vi "Main.vi"() -> ()   [LabVIEW 2020]
uses:
  Typedef/Processs.ctl
  Typedef/Low Ingregians.ctl
  Typedef/Quanities.ctl
  Assignment 14/Car Wash/CarWash/Typedefs/Queue Operations.ctl
  Typedef/DataCluster.ctl
  <vilib>/Utility/config.llb/Read Key (Boolean).vi
  <vilib>/Utility/config.llb/Write Key (Boolean).vi
  <vilib>/Utility/config.llb/NI_LVConfig.lvlib
panel:
  in  "Quantity":T1
  out "Low Ingredian":T2
  out "Process":T3
  in  "Power":bool
  out "Error Out":errorcluster
  in  "Error In":errorcluster
  out "Total Cups":dbl
  out "Elapsed Time":dbl
  out "Dispenser":dbl(slide) scale=0.0..60.0
  out "Chamber":dbl(slide) scale=0.0..60.0
  in  "Knob":i32(knob) scale=0.0..2.0
  out "Milk Level":dbl(slide)=100.0 scale=0.0..100.0
  out "Bean Level":dbl(slide)=100.0 scale=0.0..100.0
  out "Water Level":dbl(slide)=100.0 scale=0.0..100.0
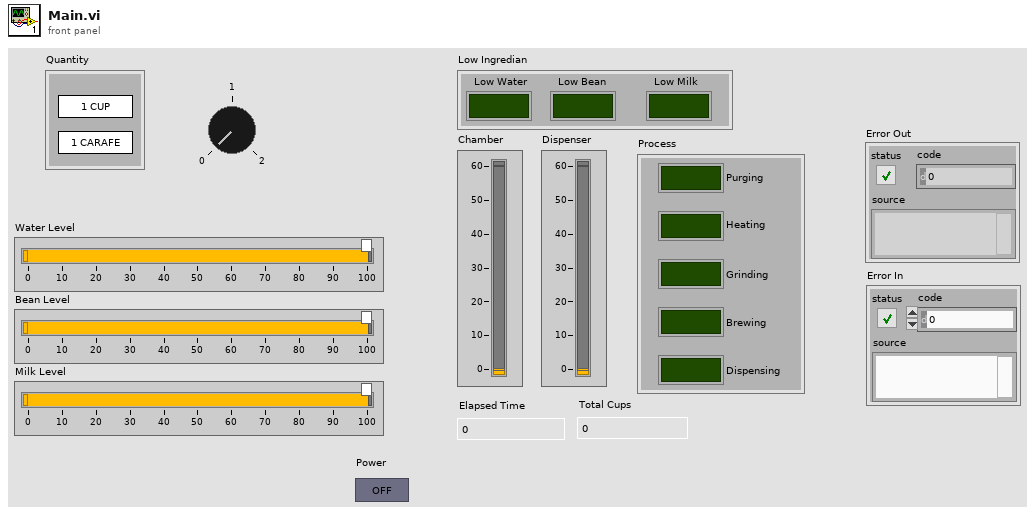
[diagram p1: front panel]
types:
  T1 = typedef "Quanities.ctl" = cluster{"1 Carafe":bool, "1 Cup":bool}
  T2 = typedef "Low Ingregians.ctl" = cluster{"Low Water":bool, "Low Bean":bool, "Low Milk":bool}
  T3 = typedef "Processs.ctl" = cluster{"Purging":bool, "Heating":bool, "Grinding":bool, "Brewing":bool, "Dispensing":bool}
  T4 = typedef "DataCluster.ctl" = cluster{"Water Level":dbl, "Bean Level":dbl, "Milk Level":dbl, "Knob":i32, "Chamber":dbl, "Dispenser":dbl, "Elapsed Time":dbl, "Total Cups":dbl, "Timer":cluster{"Previous Time":dbl, "Elapsed Time":dbl, "Start":bool, "Pause":bool, "Set Time":dbl}, "Sequence Data":i32, "Sequence":string[], "Quantity":T1, "Low Ingredian":T2, "Process":T3, "Enable array":refnum<vi>[], "Disable array":refnum<vi>[], "Power ":bool}
  T5 = typedef "Queue Operations.ctl" = enum16{"Create", "Enqueue", "Enqueue N elements", "Enstack", "Enstack N elements", "Dequeue", "Flush queue", "Release queue"}
  T6 = typedef "NI_LVConfig.lvlib/Config Data RefNum.ctl" = refnum<k1>
  T7 = enum8{"Enabled", "Disabled", "Disabled and Grayed Out"}
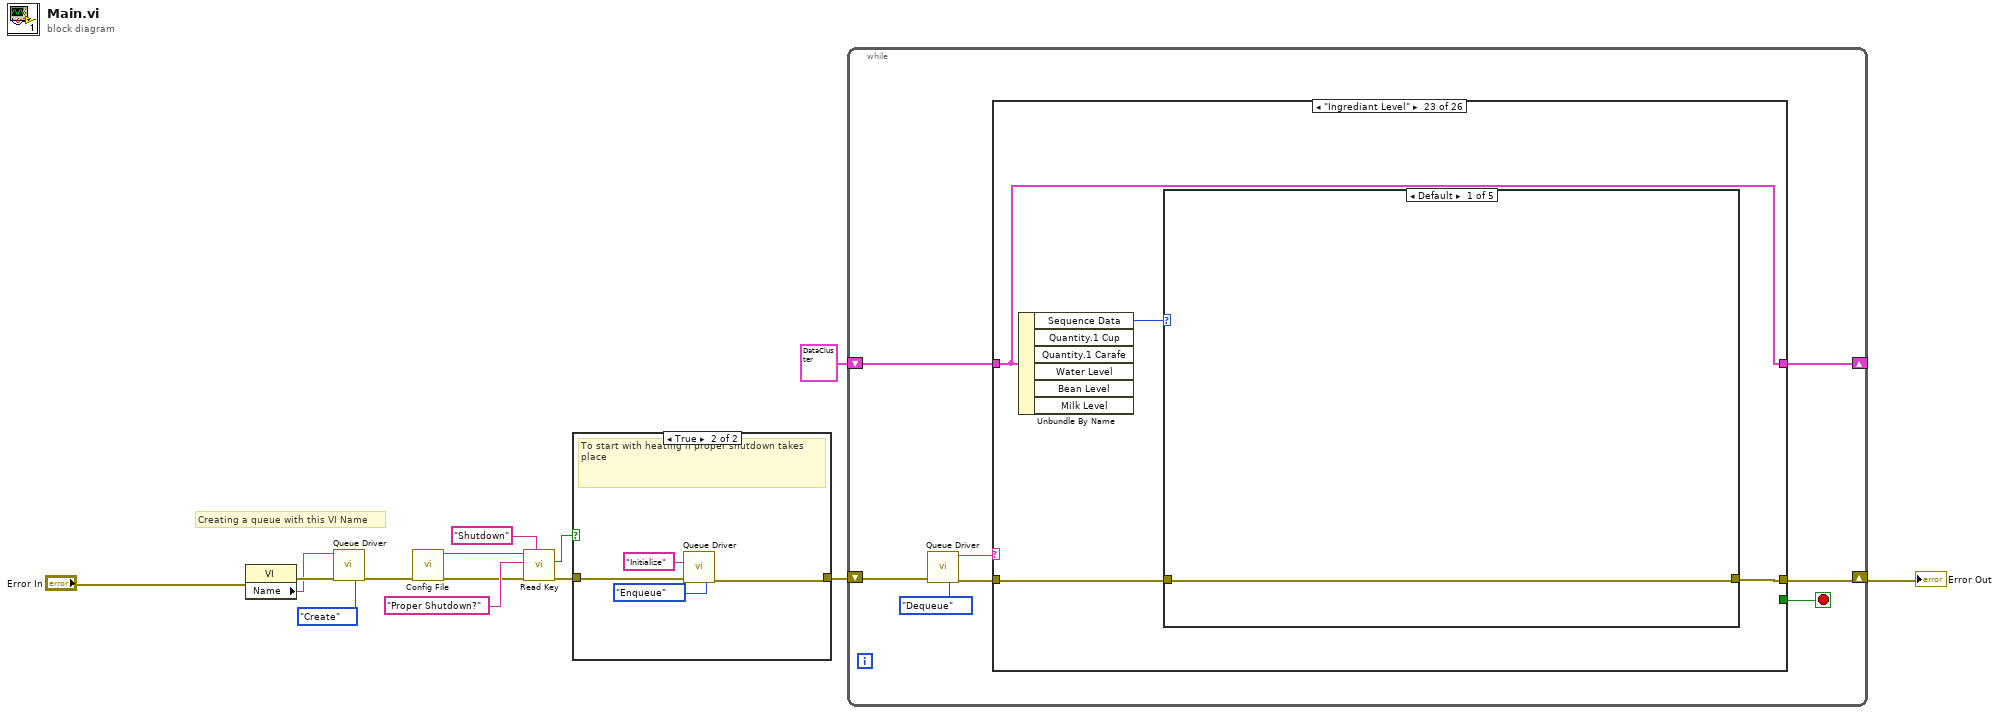
[diagram p0: block diagram]
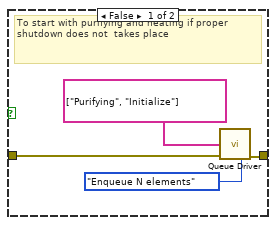
[diagram p2: hidden frame]
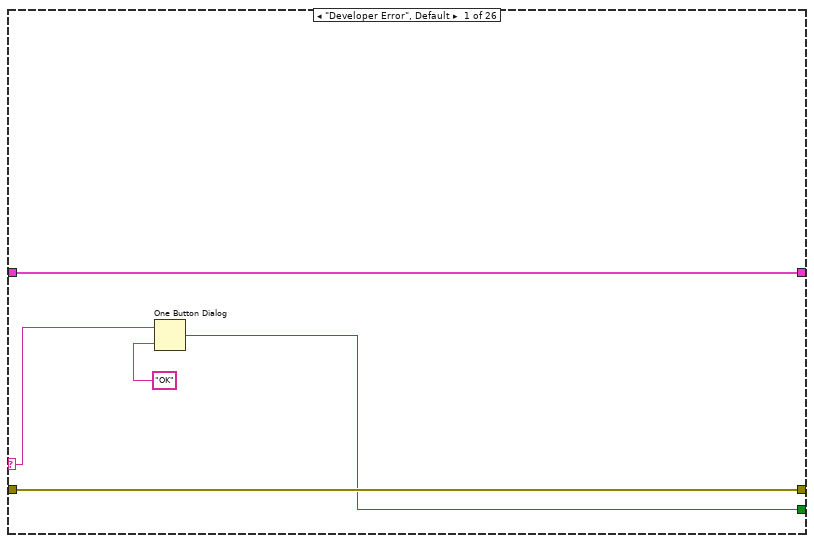
[diagram p3: hidden frame]
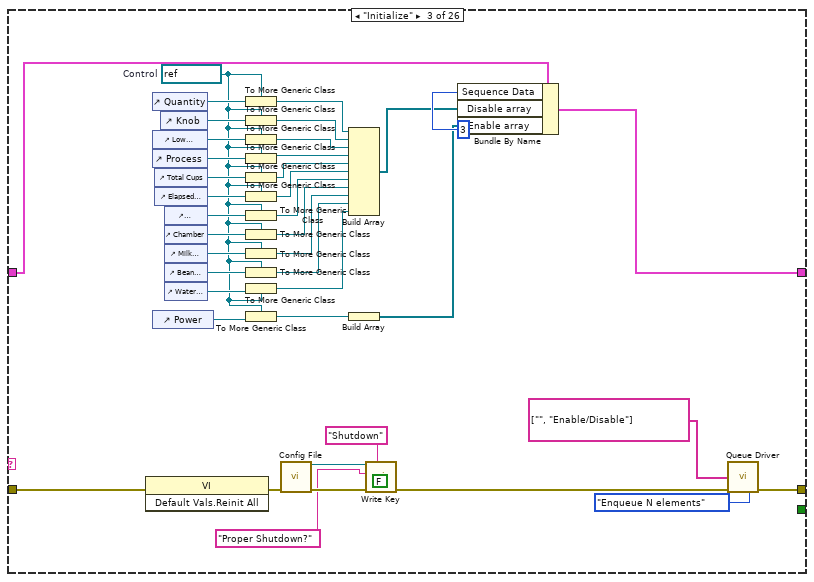
[diagram p5: hidden frame]
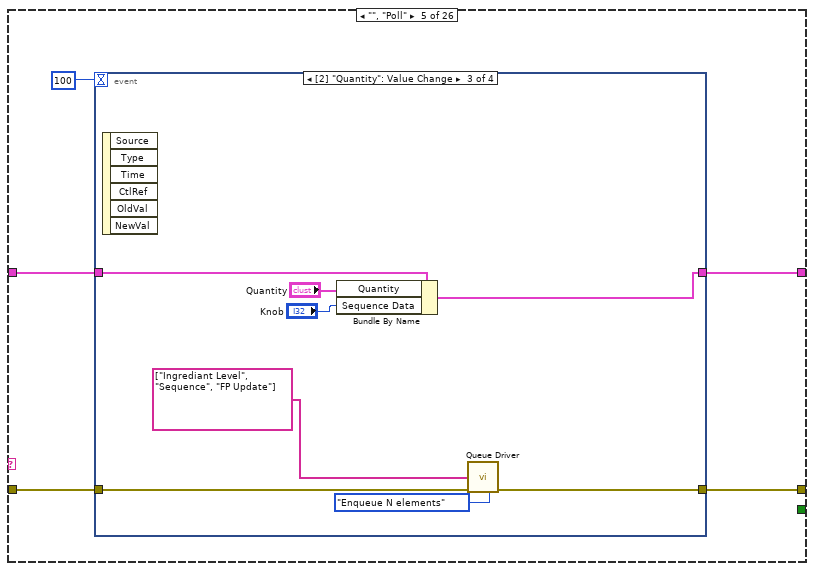
[diagram p7: hidden frame]
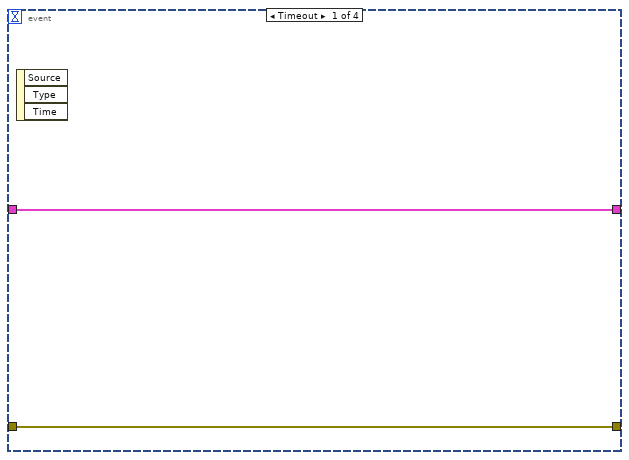
[diagram p8: hidden frame]
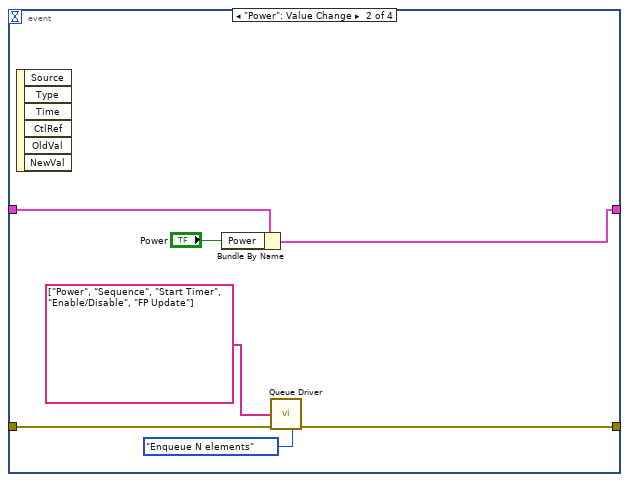
[diagram p9: hidden frame]
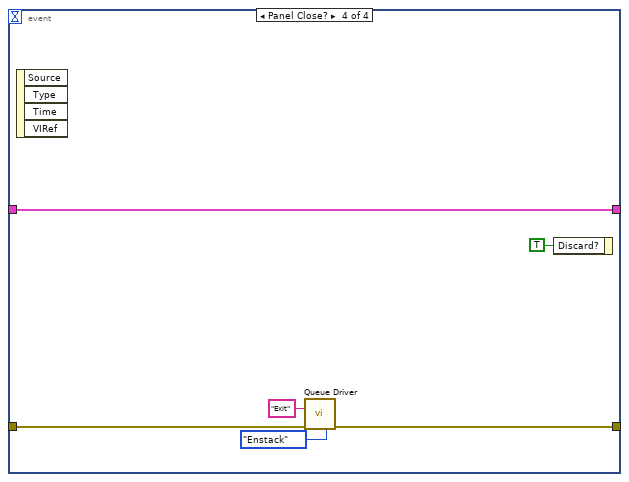
[diagram p10: hidden frame]
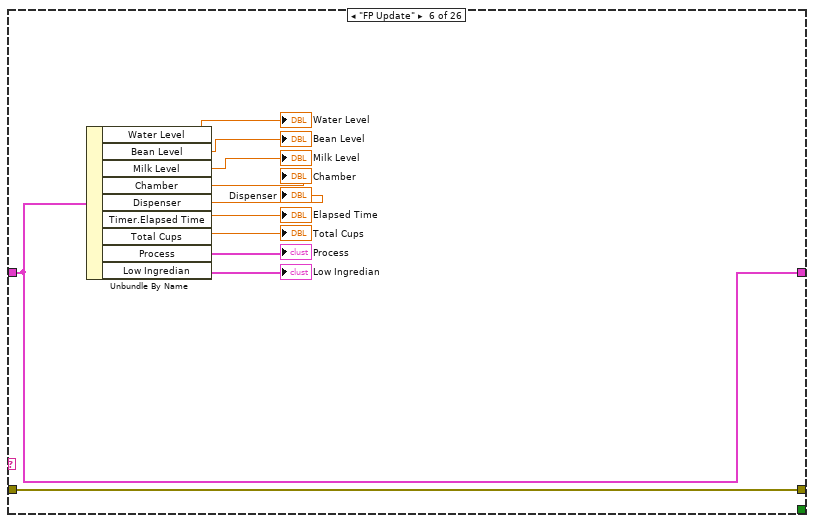
[diagram p11: hidden frame]
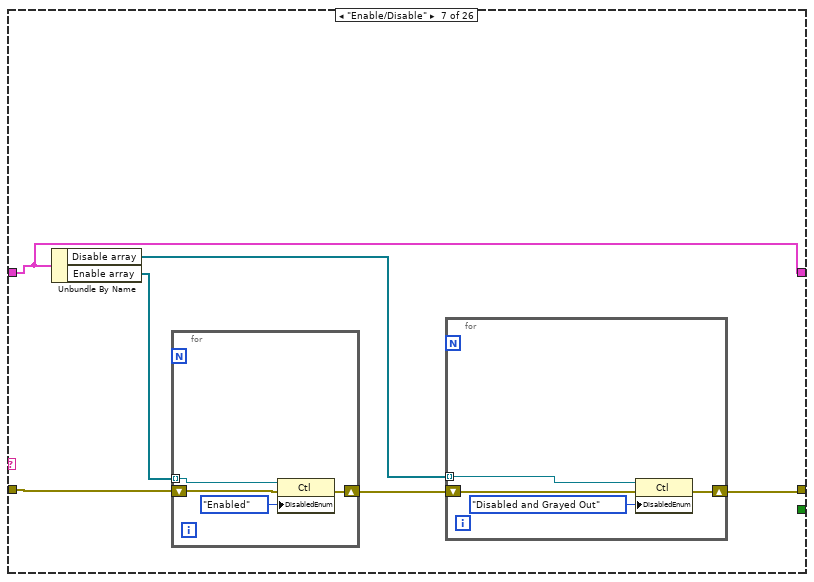
[diagram p12: hidden frame]
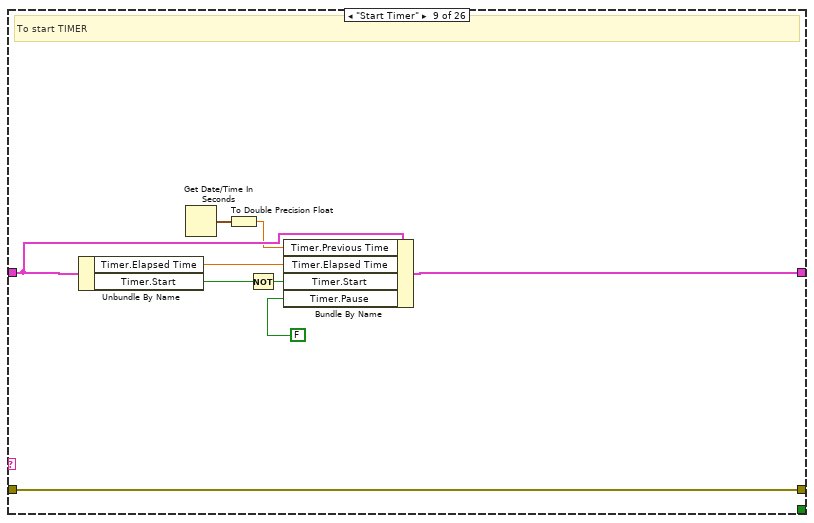
[diagram p14: hidden frame]
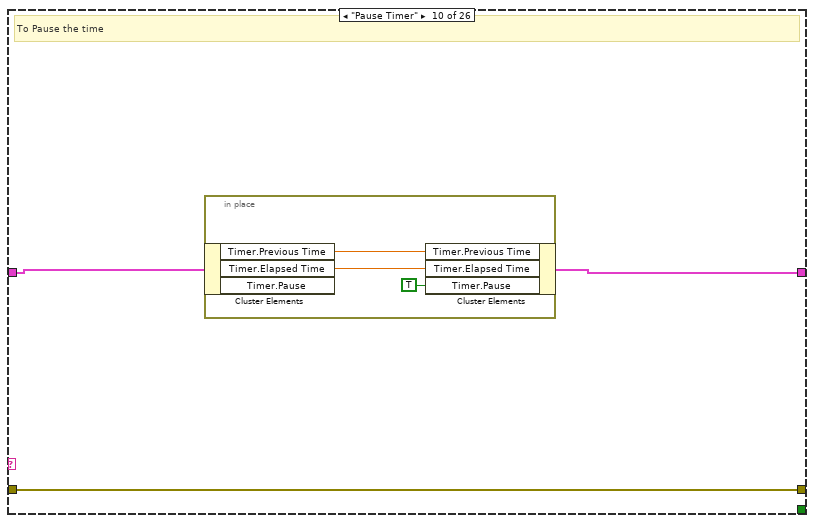
[diagram p15: hidden frame]
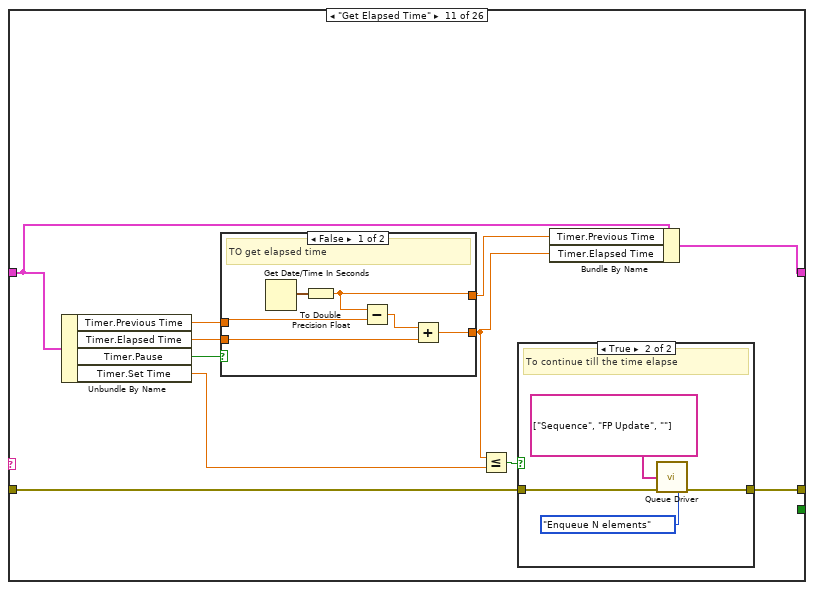
[diagram p16: hidden frame]
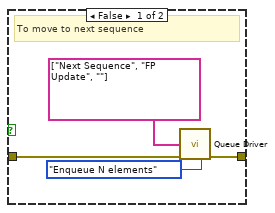
[diagram p17: hidden frame]
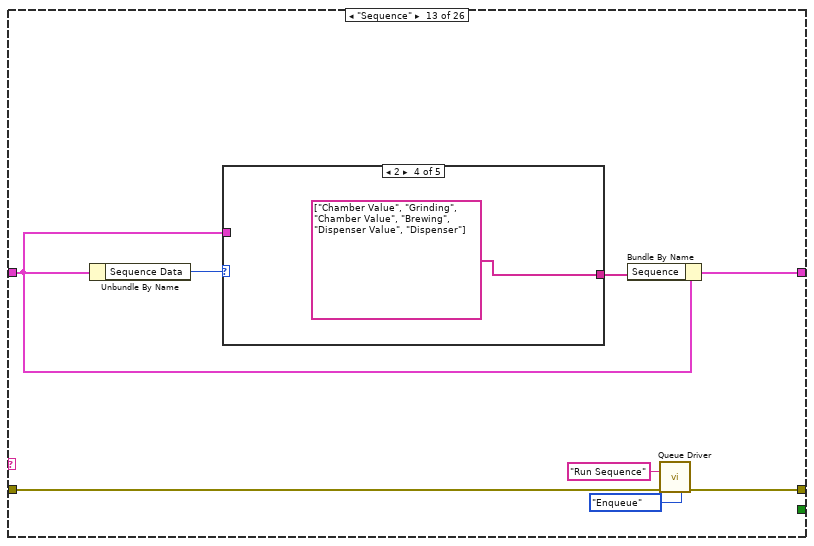
[diagram p20: hidden frame]
diagram:
  # "Creating a queue with this VI Name"
  n1 = property class="VI"(error in="Error In") -> (error out=w11:errorcluster, "Name"=w10:string)  [unwired: 1 in, 1 out]
  n2 = call "Queue Driver.vi"("Name"=w10, "Error In"=w11, "Queue operation"=Queue_Operations."Create") -> ("Error Out"=w3:errorcluster)  [unwired: 11 in, 1 out]
  n3 = call "Config File.vi"("error in"=w3) -> ("refnum"=w1:T6, "error out"=w2:errorcluster)  [unwired: 13 in]
  n4 = call-poly <vilib>:"Read Key.vi"("section"="Shutdown", "error in (no error)"=w2, "key"="Proper Shutdown?", "refnum"=w1) -> ("error out"=w7:errorcluster, "found?"=w4:bool)  [unwired: 4 in, 2 out]
  n5 = case shown="True" w4 {
    tunnel: w7 -> [w18 w22]
    tunnel: [w17 w21] -> w6
    frame False {
      # "To start with purifying and heating if proper shutdown does not  takes place"
      n6 = call "Queue Driver.vi"("Status Array"=string[] ["Purifying", "Initialize"], "Error In"=w18, "Queue operation"=Queue_Operations."Enqueue N elements") -> ("Error Out"=w17:errorcluster)  [unwired: 11 in, 1 out]
    }
    frame True {
      # "To start with heating if proper shutdown takes place"
      n7 = call "Queue Driver.vi"("Status"="Initialize", "Error In"=w22, "Queue operation"=Queue_Operations."Enqueue") -> ("Error Out"=w21:errorcluster)  [unwired: 11 in, 1 out]
    }
  }
  n8 = while {
    shift-right: [w23] -> _
    shift-left: T4 {"Water Level"=100.0, "Bean Level"=100.0, "Milk Level"=100.0, "Knob"=0, "Chamber"=0.0, "Dispenser"=0.0, "Elapsed Time"=0.0, "Total Cups"=0.0, "Timer"={"Previous Time"=0.0, "Elapsed Time"=0.0, "Start"=FALSE, "Pause"=FALSE, "Set Time"=0.0}, "Sequence Data"=0, "Sequence"=[], "Quantity"={"1 Carafe"=FALSE, "1 Cup"=FALSE}, "Low Ingredian"={"Low Water"=FALSE, "Low Bean"=FALSE, "Low Milk"=FALSE}, "Process"={"Purging"=FALSE, "Heating"=FALSE, "Grinding"=FALSE, "Brewing"=FALSE, "Dispensing"=FALSE}, "Enable array"=[], "Disable array"=[], "Power "=TRUE} ("Cluster") -> [w24]
    shift-right: [w28] -> w14
    shift-left: w6 -> [w30]
    stop <- w25 stop-if-true
    n9 = call "Queue Driver.vi"("Error In"=w30, "Queue operation"=Queue_Operations."Dequeue") -> ("Dequeued status"=w27:string, "Error Out"=w29:errorcluster)  [unwired: 12 in]
    n10 = case shown="\"Ingrediant Level\"" w27 {
      selector: w27 -> [w34 _ _ _ _ _ _ _ _ _ _ _ _ _ _ _ _ _ _ _ _ _ _ _ _ _]
      tunnel: w29 -> [w35 w37 w78 w80 w83 w112 w123 w134 w136 w145 w155 w179 w185 w199 w209 w221 w233 w245 w257 w259 w261 w263 w308 w320 w339 w345]
      tunnel: [w35 w37 w77 w80 w81 w112 w121 w134 w136 w145 w156 w179 w184 w198 w208 w220 w232 w244 w256 w259 w261 w262 w306 w315 w339 w343] -> w28
      tunnel: [w32 _ _ _ _ _ _ _ _ _ _ _ _ _ _ _ _ _ _ _ _ _ _ _ _ TRUE ("true")] -> w25
      tunnel: w24 -> [w31 w36 w74 w79 w84 w111 w120 w135 w143 w147 w153 w178 w186 w196 w202 w216 w228 w240 w252 w258 w260 w265 w305 w321 w340 w347]
      tunnel: [w31 w36 w75 w79 w82 w111 w120 w135 w142 w146 w154 w178 w180 w196 w203 w217 w229 w241 w253 w258 w260 w266 w305 w322 w340 w347] -> w23
      frame "Developer Error", Default {
        n11 = One Button Dialog(message=w34, button name ("OK")="OK") -> (true=w32:bool)
      }
      frame "/***Initialize***/" {
      }
      frame "Initialize" {
        w49 = refnum<vi> refnum  # Control
        n12 = invoke class="VI" method="Default Vals.Reinit All"(error in=w78) -> (error out=w45:errorcluster)  [unwired: 2 in, 2 out]
        n13 = control-ref of="Quantity"() -> (w72:refnum<vi>)
        n14 = control-ref of="Low Ingredian"() -> (w62:refnum<vi>)
        n15 = control-ref of="Process"() -> (w63:refnum<vi>)
        n16 = control-ref of="Power"() -> (w61:refnum<vi>)
        n17 = control-ref of="Total Cups"() -> (w64:refnum<vi>)
        n18 = control-ref of="Elapsed Time"() -> (w65:refnum<vi>)
        n19 = control-ref of="Knob"() -> (w71:refnum<vi>)
        n20 = control-ref of="Dispenser"() -> (w66:refnum<vi>)
        n21 = control-ref of="Chamber"() -> (w67:refnum<vi>)
        n22 = control-ref of="Milk Level"() -> (w68:refnum<vi>)
        n23 = control-ref of="Bean Level"() -> (w69:refnum<vi>)
        n24 = control-ref of="Water Level"() -> (w70:refnum<vi>)
        n25 = To More Generic Class(target class=w49, reference=w72) -> (generic class reference=w60:refnum<vi>)
        n26 = To More Generic Class(target class=w49, reference=w71) -> (generic class reference=w59:refnum<vi>)
        n27 = To More Generic Class(target class=w49, reference=w62) -> (generic class reference=w58:refnum<vi>)
        n28 = To More Generic Class(target class=w49, reference=w63) -> (generic class reference=w57:refnum<vi>)
        n29 = To More Generic Class(target class=w49, reference=w64) -> (generic class reference=w56:refnum<vi>)
        n30 = To More Generic Class(target class=w49, reference=w65) -> (generic class reference=w55:refnum<vi>)
        n31 = To More Generic Class(target class=w49, reference=w66) -> (generic class reference=w54:refnum<vi>)
        n32 = To More Generic Class(target class=w49, reference=w67) -> (generic class reference=w53:refnum<vi>)
        n33 = To More Generic Class(target class=w49, reference=w68) -> (generic class reference=w52:refnum<vi>)
        n34 = To More Generic Class(target class=w49, reference=w69) -> (generic class reference=w51:refnum<vi>)
        n35 = To More Generic Class(target class=w49, reference=w70) -> (generic class reference=w50:refnum<vi>)
        n36 = To More Generic Class(target class=w49, reference=w61) -> (generic class reference=w48:refnum<vi>)
        n37 = call "Config File.vi"("error in"=w45) -> ("refnum"=w42:T6, "error out"=w44:errorcluster)  [unwired: 13 in]
        n38 = Build Array(w60, w59, w58, w57, w56, w55, w54, w53, w52, w51, w50) -> (w47:refnum<vi>[])
        n39 = Build Array(w48) -> (w46:refnum<vi>[])
        n40 = call-poly <vilib>:"Write Key.vi"("section"="Shutdown", "error in (no error)"=w44, "value"=FALSE, "key"="Proper Shutdown?", "refnum"=w42) -> ("error out"=w43:errorcluster)  [unwired: 4 in, 2 out]
        n41 = Bundle By Name(cluster=w74, "Sequence Data"=3, "Disable array"=w47, "Enable array"=w46) -> (w75:T4)
        n42 = call "Queue Driver.vi"("Status Array"=string[] ["", "Enable/Disable"], "Error In"=w43, "Queue operation"=Queue_Operations."Enqueue N elements") -> ("Error Out"=w77:errorcluster)  [unwired: 11 in, 1 out]
      }
      frame "/****FP Related****/" {
      }
      frame "", "Poll" {
        n43 = event shown="[2] \"Quantity\": Value Change" {
          selector: _ -> [_ _ _ _]
          dyn-events: _ -> [_ _ _ _]
          timeout: 100 -> [_ _ _ _]
          tunnel: w84 -> [w87 w93 w102 w104]
          tunnel: w83 -> [w86 w91 w99 w108]
          tunnel: [w87 w94 w101 w104] -> w82
          tunnel: [w86 w90 w98 w107] -> w81
          event Timeout {
            n44 = event-data() -> ()  [unwired: 1 in, 3 out]
          }
          event "Power": Value Change {
            n45 = event-data() -> ()  [unwired: 1 in, 6 out]
            n46 = Bundle By Name(cluster=w93, "Power"="Power") -> (w94:T4)
            n47 = call "Queue Driver.vi"("Status Array"=string[] ["Power", "Sequence", "Start Timer", "Enable/Disable", "FP Update"], "Error In"=w91, "Queue operation"=Queue_Operations."Enqueue N elements") -> ("Error Out"=w90:errorcluster)  [unwired: 11 in, 1 out]
          }
          event Value Change {
            n48 = event-data() -> ()  [unwired: 1 in, 6 out]
            n49 = Bundle By Name(cluster=w102, "Quantity"="Quantity", "Sequence Data"="Knob") -> (w101:T4)
            n50 = call "Queue Driver.vi"("Status Array"=string[] ["Ingrediant Level", "Sequence", "FP Update"], "Error In"=w99, "Queue operation"=Queue_Operations."Enqueue N elements") -> ("Error Out"=w98:errorcluster)  [unwired: 11 in, 1 out]
          }
          event Panel Close? {
            n51 = event-data() -> ()  [unwired: 1 in, 4 out]
            n52 = call "Queue Driver.vi"("Status"="Exit", "Error In"=w108, "Queue operation"=Queue_Operations."Enstack") -> ("Error Out"=w107:errorcluster)  [unwired: 11 in, 1 out]
            n53 = event-data("Discard?"=TRUE) -> ()  [unwired: 1 in, 1 out]
          }
        }
      }
      frame "FP Update" {
        n54 = Unbundle By Name(w111) -> ("Water Level"=→"Water Level":dbl, "Bean Level"=→"Bean Level":dbl, "Milk Level"=→"Milk Level":dbl, "Chamber"=→"Chamber":dbl, "Dispenser"=→"Dispenser":dbl, "Timer.Elapsed Time"=→"Elapsed Time":dbl, "Total Cups"=→"Total Cups":dbl, "Process"=→"Process":T3, "Low Ingredian"=→"Low Ingredian":T2)
      }
      frame "Enable/Disable" {
        n55 = Unbundle By Name(w120) -> ("Disable array"=w124:refnum<vi>[], "Enable array"=w125:refnum<vi>[])
        n56 = for {
          tunnel: w125 -> [w133] mode=indexing
          shift-right: [w130] -> w122
          shift-left: w123 -> [w131]
          n57 = property class="Ctl"(reference=w133, error in=w131, "DisabledEnum"=T7."Enabled" ("Disabled")) -> (error out=w130:errorcluster)  [unwired: 1 out]
        }
        n58 = for {
          tunnel: w124 -> [w127] mode=indexing
          shift-right: [w128] -> w121
          shift-left: w122 -> [w129]
          n59 = property class="Ctl"(reference=w127, error in=w129, "DisabledEnum"=T7."Disabled and Grayed Out" ("Disabled")) -> (error out=w128:errorcluster)  [unwired: 1 out]
        }
      }
      frame "/****Timer****/" {
      }
      frame "Start Timer" {
        # "To start TIMER"
        n60 = Unbundle By Name(w143) -> ("Timer.Elapsed Time"=w140:dbl, "Timer.Start"=w138:bool)
        n61 = Get Date/Time In Seconds() -> (seconds since 1Jan1904=w144:timestamp)
        n62 = To Double Precision Float(number=w144) -> (double precision float=w141:dbl)
        n63 = Not(x=w138) -> (.not. x?=w137:bool)
        n64 = Bundle By Name(cluster=w143, "Timer.Previous Time"=w141, "Timer.Elapsed Time"=w140, "Timer.Start"=w137, "Timer.Pause"=FALSE) -> (w142:T4)
      }
      frame "Pause Timer" {
        # "To Pause the time"
        n65 = in-place {
          n66 = in-place-cluster #1(w147) -> ("Timer.Previous Time"=w150:dbl, "Timer.Elapsed Time"=w149:dbl)  [unwired: 1 out]
          n67 = in-place-cluster #1("Timer.Previous Time"=w150, "Timer.Elapsed Time"=w149, "Timer.Pause"=TRUE) -> (w146:T4)
        }
      }
      frame "Get Elapsed Time" {
        n68 = Unbundle By Name(w153) -> ("Timer.Previous Time"=w159:dbl, "Timer.Elapsed Time"=w160:dbl, "Timer.Pause"=w161:bool, "Timer.Set Time"=w158:dbl)
        n69 = case shown="False" w161 {
          tunnel: w160 -> [w172 w176]
          tunnel: w159 -> [w174 w177]
          tunnel: [w171 w176] -> w151
          tunnel: [w170 w177] -> w152
          frame False {
            # "TO get elapsed time"
            n70 = Get Date/Time In Seconds() -> (seconds since 1Jan1904=w175:timestamp)
            n71 = To Double Precision Float(number=w175) -> (double precision float=w170:dbl)
            n72 = Subtract(x=w170, y=w174) -> (x-y=w173:dbl)
            n73 = Add(x=w173, y=w172) -> (x+y=w171:dbl)
          }
          frame True {
            # "To paused time"
          }
        }
        n74 = Less Or Equal?(x=w151, y=w158) -> (x <= y?=w157:bool)
        n75 = case shown="True" w157 {
          tunnel: [w164 w169] -> w156
          tunnel: w155 -> [w165 w168]
          frame False {
            # "To move to next sequence"
            n76 = call "Queue Driver.vi"("Status Array"=string[] ["Next Sequence", "FP Update", ""], "Error In"=w165, "Queue operation"=Queue_Operations."Enqueue N elements") -> ("Error Out"=w164:errorcluster)  [unwired: 11 in, 1 out]
          }
          frame True {
            # "To continue till the time elapse"
            n77 = call "Queue Driver.vi"("Status Array"=string[] ["Sequence", "FP Update", ""], "Error In"=w168, "Queue operation"=Queue_Operations."Enqueue N elements") -> ("Error Out"=w169:errorcluster)  [unwired: 11 in, 1 out]
          }
        }
        n78 = Bundle By Name(cluster=w153, "Timer.Previous Time"=w152, "Timer.Elapsed Time"=w151) -> (w154:T4)
      }
      frame "/****Functionalities***/" {
      }
      frame "Sequence" {
        n79 = Unbundle By Name(w186) -> ("Sequence Data"=w187:i32)
        n80 = case shown="2" w187 {
          tunnel: w186 -> [_ _ _ _ _]
          tunnel: [string[] [] ("Sequence") string[] ["Dispenser", "Dispenser Value"] ("Sequence") string[] ["Chamber Value", "Grinding", "Chamber Value", "Brewing", "Dispenser Value", "Dispenser"] ("Sequence") string[] ["Chamber Value", "Grinding", "Chamber Value", "Brewing", "Dispenser Value", "Dispenser"] ("Sequence") string[] ["Heating"] ("Sequence")] -> w181
          frame Default {
          }
          frame 0 {
          }
          frame 1 {
          }
          frame 2 {
          }
          frame 3 {
          }
        }
        n81 = Bundle By Name(cluster=w186, "Sequence"=w181) -> (w180:T4)
        n82 = call "Queue Driver.vi"("Status"="Run Sequence", "Error In"=w185, "Queue operation"=Queue_Operations."Enqueue") -> ("Error Out"=w184:errorcluster)  [unwired: 11 in, 1 out]
      }
      frame "Run Sequence" {
        n83 = Unbundle By Name(w196) -> ("Sequence"=w195:string[])
        n84 = Delete From Array(array=w195, index=0) -> (deleted portion=w193:string)  [unwired: 1 in, 1 out]
        n85 = call "Queue Driver.vi"("Status"=w193, "Error In"=w199, "Queue operation"=Queue_Operations."Enqueue") -> ("Error Out"=w198:errorcluster)  [unwired: 11 in, 1 out]
      }
      frame "Next Sequence" {
        n86 = Unbundle By Name(w202) -> ("Sequence"=w206:string[])
        n87 = Delete From Array(array=w206, index=0) -> (array with subset deleted=w204:string[])  [unwired: 1 in, 1 out]
        n88 = Bundle By Name(cluster=w202, "Sequence"=w204, "Timer.Elapsed Time"=0.0) -> (w203:T4)
        n89 = call "Queue Driver.vi"("Status Array"=string[] ["Run Sequence"], "Error In"=w209, "Queue operation"=Queue_Operations."Enqueue N elements") -> ("Error Out"=w208:errorcluster)  [unwired: 11 in, 1 out]
      }
      frame "Heating" {
        # "To make heat glow for 5 sec initially"
        n90 = Bundle By Name(cluster=w216, "Timer.Set Time"=5.0, "Process.Purging"=FALSE ("Purging"), "Process.Heating"=TRUE ("Heating"), "Process.Grinding"=FALSE ("Grinding"), "Process.Brewing"=FALSE ("Brewing"), "Process.Dispensing"=FALSE ("Dispensing")) -> (w217:T4)
        n91 = call "Queue Driver.vi"("Status Array"=string[] ["Get Elapsed Time", "FP Update"], "Error In"=w221, "Queue operation"=Queue_Operations."Enqueue N elements") -> ("Error Out"=w220:errorcluster)  [unwired: 11 in, 1 out]
      }
      frame "Dispenser" {
        # "Time taken to dispense"
        n92 = Bundle By Name(cluster=w228, "Timer.Set Time"=5.0, "Process.Purging"=FALSE ("Purging"), "Process.Heating"=FALSE ("Heating"), "Process.Grinding"=FALSE ("Grinding"), "Process.Brewing"=FALSE ("Brewing"), "Process.Dispensing"=TRUE ("Dispensing")) -> (w229:T4)
        n93 = call "Queue Driver.vi"("Status Array"=string[] ["Get Elapsed Time", "FP Update"], "Error In"=w233, "Queue operation"=Queue_Operations."Enqueue N elements") -> ("Error Out"=w232:errorcluster)  [unwired: 11 in, 1 out]
      }
      frame "Grinding" {
        # "Time taken to grind after the bean is taken as input"
        n94 = Bundle By Name(cluster=w240, "Timer.Set Time"=3.0, "Process.Purging"=FALSE ("Purging"), "Process.Heating"=FALSE ("Heating"), "Process.Grinding"=TRUE ("Grinding"), "Process.Brewing"=FALSE ("Brewing"), "Process.Dispensing"=FALSE ("Dispensing")) -> (w241:T4)
        n95 = call "Queue Driver.vi"("Status Array"=string[] ["Get Elapsed Time", "FP Update"], "Error In"=w245, "Queue operation"=Queue_Operations."Enqueue N elements") -> ("Error Out"=w244:errorcluster)  [unwired: 11 in, 1 out]
      }
      frame "Brewing" {
        # "Time taken for brewing"
        n96 = Bundle By Name(cluster=w252, "Timer.Set Time"=4.0, "Process.Purging"=FALSE ("Purging"), "Process.Heating"=FALSE ("Heating"), "Process.Grinding"=FALSE ("Grinding"), "Process.Brewing"=TRUE ("Brewing"), "Process.Dispensing"=FALSE ("Dispensing")) -> (w253:T4)
        n97 = call "Queue Driver.vi"("Status Array"=string[] ["Get Elapsed Time", "FP Update"], "Error In"=w257, "Queue operation"=Queue_Operations."Enqueue N elements") -> ("Error Out"=w256:errorcluster)  [unwired: 11 in, 1 out]
      }
      frame "Chamber Value" {
        # "The chamber value will be updating once the coffee preparation starts and the value of bean, waterand milk will be added to this chamber to indicate the ingredients amount"
      }
      frame "Dispenser Value" {
        # "It will display the dispensing amount in diplay while dispensing"
      }
      frame "Power" {
        w269 = refnum<vi> refnum  # Control
        # "Once the power on all the controls should be enabled"
        n98 = Unbundle By Name(w265) -> ("Power"=w264:bool)
        n99 = control-ref of="Quantity"() -> (w293:refnum<vi>)
        n100 = control-ref of="Low Ingredian"() -> (w283:refnum<vi>)
        n101 = control-ref of="Process"() -> (w284:refnum<vi>)
        n102 = control-ref of="Power"() -> (w282:refnum<vi>)
        n103 = control-ref of="Total Cups"() -> (w285:refnum<vi>)
        n104 = control-ref of="Elapsed Time"() -> (w286:refnum<vi>)
        n105 = control-ref of="Knob"() -> (w292:refnum<vi>)
        n106 = control-ref of="Dispenser"() -> (w287:refnum<vi>)
        n107 = control-ref of="Chamber"() -> (w288:refnum<vi>)
        n108 = control-ref of="Milk Level"() -> (w289:refnum<vi>)
        n109 = control-ref of="Bean Level"() -> (w290:refnum<vi>)
        n110 = control-ref of="Water Level"() -> (w291:refnum<vi>)
        n111 = To More Generic Class(target class=w269, reference=w293) -> (generic class reference=w281:refnum<vi>)
        n112 = To More Generic Class(target class=w269, reference=w292) -> (generic class reference=w280:refnum<vi>)
        n113 = To More Generic Class(target class=w269, reference=w283) -> (generic class reference=w279:refnum<vi>)
        n114 = To More Generic Class(target class=w269, reference=w284) -> (generic class reference=w278:refnum<vi>)
        n115 = To More Generic Class(target class=w269, reference=w285) -> (generic class reference=w277:refnum<vi>)
        n116 = To More Generic Class(target class=w269, reference=w286) -> (generic class reference=w276:refnum<vi>)
        n117 = To More Generic Class(target class=w269, reference=w287) -> (generic class reference=w275:refnum<vi>)
        n118 = To More Generic Class(target class=w269, reference=w288) -> (generic class reference=w274:refnum<vi>)
        n119 = To More Generic Class(target class=w269, reference=w289) -> (generic class reference=w273:refnum<vi>)
        n120 = To More Generic Class(target class=w269, reference=w290) -> (generic class reference=w272:refnum<vi>)
        n121 = To More Generic Class(target class=w269, reference=w282) -> (generic class reference=w270:refnum<vi>)
        n122 = To More Generic Class(target class=w269, reference=w291) -> (generic class reference=w271:refnum<vi>)
        n123 = case shown="False" w264 {
          tunnel: w263 -> [w303 w304]
          tunnel: [w295 w304] -> w262
          frame False {
            n124 = call "Queue Driver.vi"("Status"="Exit", "Error In"=w303, "Queue operation"=Queue_Operations."Enstack") -> ("Error Out"=w300:errorcluster)  [unwired: 11 in, 1 out]
            n125 = call "Config File.vi"("error in"=w300) -> ("refnum"=w294:T6, "error out"=w299:errorcluster)  [unwired: 13 in]
            n126 = call-poly <vilib>:"Write Key.vi"("section"="Shutdown", "error in (no error)"=w299, "value"=TRUE, "key"="Proper Shutdown?", "refnum"=w294) -> ("error out"=w295:errorcluster)  [unwired: 4 in, 2 out]
          }
          frame True {
          }
        }
        n127 = Build Array(w281, w280, w279, w278, w277, w276, w275, w274, w273, w272, w271, w270) -> (w268:refnum<vi>[])
        n128 = Bundle By Name(cluster=w265, "Enable array"=w268, "Disable array"=refnum<vi>[] []) -> (w266:T4)
      }
      frame "Ingrediant Level" {
        n129 = Unbundle By Name(w305) -> ("Sequence Data"=w307:i32)  [unwired: 5 out]
        n130 = case shown="Default" w307 {
          tunnel: w308 -> [w309 w310 w311 w312 w313]
          tunnel: [w309 w310 w311 w312 w313] -> w306
          frame Default {
          }
          frame 0 {
          }
          frame 1 {
          }
          frame 2 {
          }
          frame 3 {
          }
        }
      }
      frame "Ingrediant Indicator" {
        w323 = 30.0
        n131 = Unbundle By Name(w321) -> ("Water Level"=w326:dbl, "Bean Level"=w325:dbl, "Milk Level"=w324:dbl)
        n132 = Less?(x=w326, y=w323) -> (x < y?=w314:bool)
        n133 = Less?(x=w325, y=w323) -> (x < y?=w317:bool)
        n134 = Less?(x=w324, y=w323) -> (x < y?=w319:bool)
        n135 = case shown="False" w319 {
          tunnel: w320 -> [w335 w338]
          tunnel: [w335 w337] -> w318
          frame False {
          }
          frame True {
            n136 = property on="Knob" class="Knob (strict)"(error in=w338, "Maximum"=1.0 ("Data Entry Limits:Maximum")) -> (error out=w337:errorcluster)  [unwired: 1 in, 1 out]
          }
        }
        n137 = case shown="False" w317 {
          tunnel: w318 -> [w331 w334]
          tunnel: [w331 w333] -> w316
          frame False {
          }
          frame True {
            n138 = property on="Knob" class="Knob (strict)"(error in=w334, "Maximum"=1.0 ("Data Entry Limits:Maximum")) -> (error out=w333:errorcluster)  [unwired: 1 in, 1 out]
          }
        }
        n139 = case shown="False" w314 {
          tunnel: w316 -> [w327 w330]
          tunnel: [w327 w329] -> w315
          frame False {
          }
          frame True {
            n140 = property on="Knob" class="Knob (strict)"(error in=w330, "DisabledEnum"=T7."Enabled" ("Disabled")) -> (error out=w329:errorcluster)  [unwired: 1 in, 1 out]
          }
        }
        n141 = Bundle By Name(cluster=w321, "Low Ingredian.Low Water"=w314, "Low Ingredian.Low Bean"=w317, "Low Ingredian.Low Milk"=w319) -> (w322:T4)
      }
      frame "/***Exit***/" {
      }
      frame "Exit" {
        n142 = call "Queue Driver.vi"("Error In"=w345, "Queue operation"=Queue_Operations."Flush queue") -> ("Error Out"=w344:errorcluster)  [unwired: 12 in, 1 out]
        n143 = call "Queue Driver.vi"("Error In"=w344, "Queue operation"=Queue_Operations."Release queue") -> ("Error Out"=w343:errorcluster)  [unwired: 12 in, 1 out]
      }
    }
  }
  "Error Out" <- w14
